vi "Perform Action.vi"(8 "error in":errorcluster, 10 "Input":variant, 11 "DIO DAQmx Fixed Freq PWM CFG in":refnum<class "CO DAQmx Fixed Freq PWM CFG.lvclass">) -> (0 "error out":errorcluster, 2 "Output":variant, 3 "DIO DAQmx Fixed Freq PWM CFG out":refnum<class "CO DAQmx Fixed Freq PWM CFG.lvclass">)   [LabVIEW 2023, in "CO DAQmx Fixed Freq PWM CFG.lvclass"]
uses:
  CO DAQmx Fixed Freq PWM CFG.lvclass
  DAQmx Base CFG/DAQmx Base CFG.lvclass/DAQmx Base CFG.ctl
  <resource>/objmgr/daqmx.rc
  DAQmx Base CFG/DAQmx Base CFG.lvclass
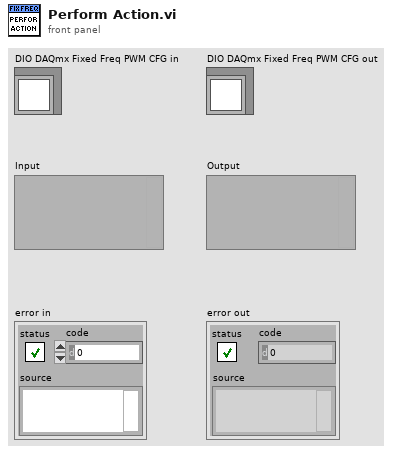
[diagram p1: front panel]
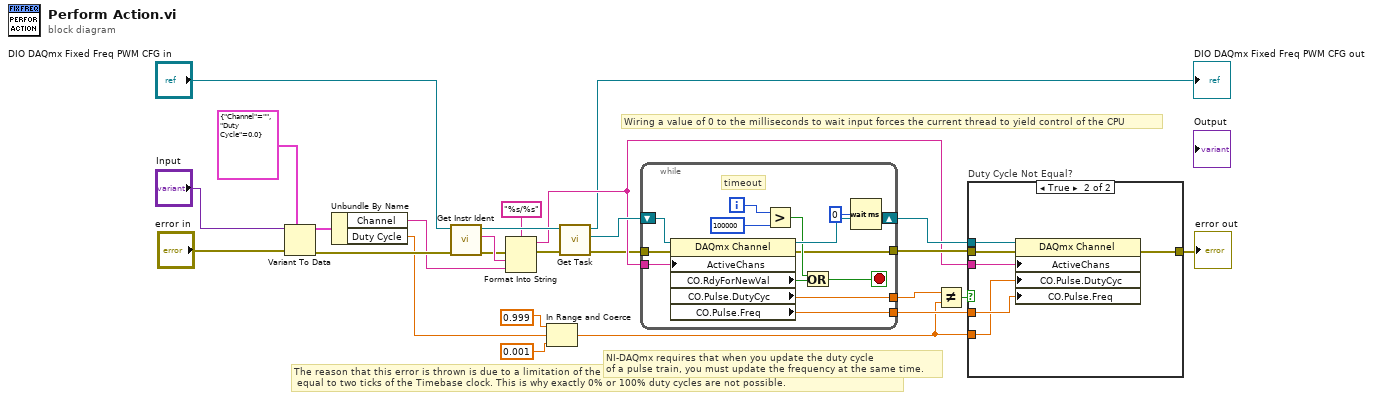
[diagram p0: block diagram]
diagram:
  # "The reason that this error is thrown is due to a limitation of the DAQ devices: the minimum duty cycle that can be set is\n equal to two ticks of the Timebase clock. This is why exactly 0% or 100% duty cycles are not possible."
  # "Wiring a value of 0 to the milliseconds to wait input forces the current thread to yield control of the CPU"
  # "NI-DAQmx requires that when you update the duty cycle\nof a pulse train, you must update the frequency at the same time."
  n1 = Variant To Data(error in="error in", type=cluster{"Channel":string, "Duty Cycle":dbl} {"Channel"="", "Duty Cycle"=0.0}, Variant="Input") -> (data=w23:cluster{"Channel":string, "Duty Cycle":dbl}, error out=w24:errorcluster)
  n2 = Unbundle By Name(w23) -> ("Channel"=w19:string, "Duty Cycle"=w11:dbl)
  n3 = call-dynamic "Get Instr Ident.vi"("error in"=w24, "CFG JSON in"="DIO DAQmx Fixed Freq PWM CFG in") -> ("error out"=w18:errorcluster, "Instr Ident"=w20:string, "CFG JSON out"=w22:refnum<class "CO DAQmx Fixed Freq PWM CFG.lvclass">)  [unwired: 7 in]
  n4 = Format Into String(format string="%s/%s", error in=w18, w20, w19) -> (resulting string=w13:string, error out=w2:errorcluster)  [unwired: 1 in]
  n5 = In Range and Coerce(upper limit=0.999, x=w11, lower limit=0.001) -> (coerced(x)=w5:dbl)  [unwired: 1 out]
  n6 = call "Get Task.vi"("DAQmx Base CFG in"=w22) -> ("Task"=w15:refnum<k21>, "DAQmx Base CFG out"=→"DIO DAQmx Fixed Freq PWM CFG out":refnum<class "CO DAQmx Fixed Freq PWM CFG.lvclass">)  [unwired: 9 in]
  n7 = while {
    tunnel: [w37] -> w10
    tunnel: w2 -> [w36]
    tunnel: [w34] -> w12
    tunnel: w13 -> [w33]
    shift-right: [w38] -> w17
    shift-left: w15 -> [w35]
    tunnel: [w26] -> w14
    i -> [w31]
    stop <- w29 stop-if-true
    # "timeout"
    n8 = property class="DAQmx Channel"(reference=w35, error in=w36, "ActiveChans"=w33) -> (reference out=w38:refnum<k21>, error out=w26:errorcluster, "CO.RdyForNewVal"=w32:bool, "CO.Pulse.DutyCyc"=w37:dbl, "CO.Pulse.Freq"=w34:dbl)
    n9 = Greater?(x=w31, y=100000) -> (0:w28:bool)
    n10 = Or(x=w28, y=w32) -> (x .or. y?=w29:bool)
    n11 = Wait (ms)(milliseconds to wait=u32 0) -> ()  [unwired: 1 out]
  }
  n12 = Not Equal?(x=w10, y=w5) -> (x != y?=w16:bool)
  n13 = case "Duty Cycle Not Equal?" shown="True" w16 {
    tunnel: [w39 w45] -> w6
    tunnel: w14 -> [w39 w44]
    tunnel: w17 -> [_ w43]
    tunnel: w13 -> [_ w42]
    tunnel: w12 -> [_ w41]
    tunnel: w5 -> [_ w40]
    frame False {
    }
    frame True {
      n14 = property class="DAQmx Channel"(reference=w43, error in=w44, "ActiveChans"=w42, "CO.Pulse.DutyCyc"=w40, "CO.Pulse.Freq"=w41) -> (error out=w45:errorcluster)  [unwired: 1 out]
    }
  }
  "error out" <- w6
